vi "io.xor.vi"(8 "error in":errorcluster, 10 "Start Index (0)":u8, 11 "payload in":string) -> (0 "error out":errorcluster, 1 "Xor(payload) num":u8, 2 "XOR(payload)":string)   [LabVIEW 2024]
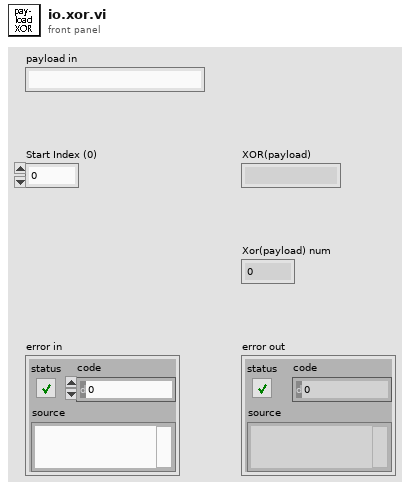
[diagram p1: front panel]
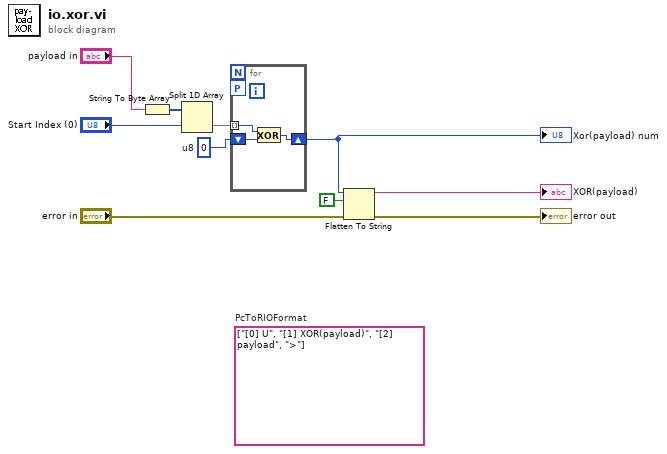
[diagram p0: block diagram]
diagram:
  (unwired) string[] ["[0] U", "[1] XOR(payload)", "[2] payload", ">"]  # PcToRIOFormat
  w5 = u8 0  # u8
  n1 = String To Byte Array(string="payload in") -> (unsigned byte array=w7:u8[])
  n2 = Split 1D Array(array=w7, index="Start Index (0)") -> (second subarray=w9:u8[])  [unwired: 1 out]
  n3 = for {
    tunnel: w9 -> [w13] mode=indexing
    shift-right: [w12] -> w4
    shift-left: w5 -> [w11]
    workers-P: _ -> [_]
    n4 = Exclusive Or(1:w11, 2:w13) -> (0:w12:u8)
  }
  "Xor(payload) num" <- w4
  n5 = Flatten To String(anything=w4, prepend array or string size? (T)=FALSE, error in (no error)="error in") -> (data string=→"XOR(payload)":string, error out=→"error out":errorcluster)  [unwired: 1 in, 1 out]
